vi "miniScanSelector.vi"(0 "X-Y-Z coordinates":T1 {"Apparent Frame Size" format="%#_6f"; "Original FOV (um)" format="%#_6f"; "Pixels per miniscan" format="%#_6f"; "Dwell Time per pixel" format="%#_6f"; "Resolution" format="%#_6f"; "ROI group ID" format="%#_6f"; "Laser Power (%)" format="%#_6f"; "Zoom" format="%#_6f"; "Frame Size" format="%#_6f"; "Number of lines" format="%#_6f"; "Composite ID" format="%#_6f"; "Angle (deg)" format="%#_6f"; "ROI Time (ns)" format="%#_6f"; "ROI ID" format="%#_6f"; "Pixels in ROI" format="%#_6f"; "ROI index" format="%#_6f"; "Z stop" format="%#_6f"; "Y stop" format="%#_6f"; "X stop" format="%#_6f"; "Z start" format="%#_6f"; "X start" format="%#_6f"; "Y start" format="%#_6f"}, 1 "index":i32, 2 "FrameSize":dbl, 3 "App. FrameSize":dbl, 5 "Main zoom":dbl) -> (14 "Norm X Start":dbl, 15 "Norm Y Start":dbl, 16 "Norm Z Start":dbl, 17 "Norm X Stop":dbl, 18 "Norm Y Stop":dbl, 19 "Norm Z Stop":dbl)   [LabVIEW 2020]
uses:
  User Interface/Visualisation/Functional Imaging Viewer/Typedefs/ROI parameters data type.ctl
panel:
  in  "Temporary offset (0)":dbl format="%#_13g"
  # "<--- For vertical miniscans only"
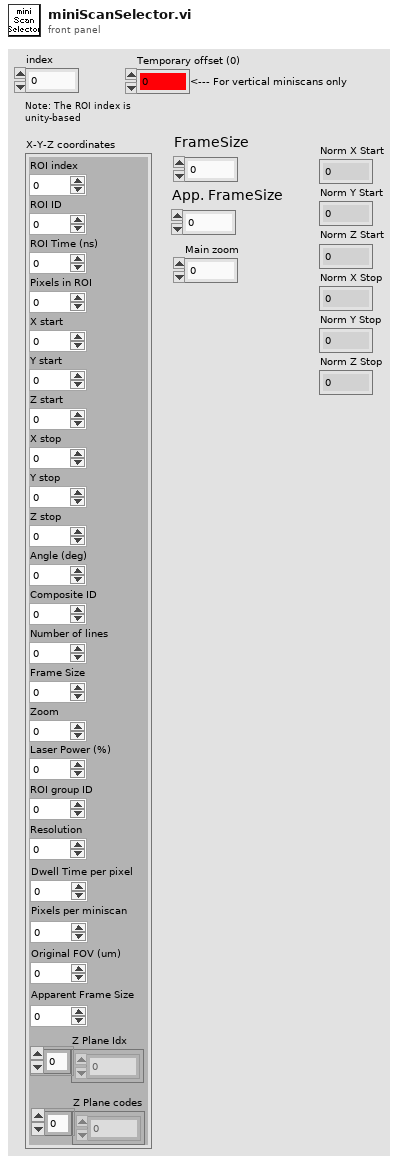
[diagram p1: front panel]
types:
  T1 = typedef "ROI parameters data type.ctl" = cluster{"ROI index":dbl, "ROI ID":dbl, "ROI Time (ns)":dbl, "Pixels in ROI":dbl, "X start":dbl, "Y start":dbl, "Z start":dbl, "X stop":dbl, "Y stop":dbl, "Z stop":dbl, "Angle (deg)":dbl, "Composite ID":dbl, "Number of lines":dbl, "Frame Size":dbl, "Zoom":dbl, "Laser Power (%)":dbl, "ROI group ID":dbl, "Resolution":dbl, "Dwell Time per pixel":dbl, "Pixels per miniscan":dbl, "Original FOV (um)":dbl, "Apparent Frame Size":dbl, "Z Plane Idx":i32[], "Z Plane codes":i32[]}
  T2 = typedef "Angle type.ctl" = enum16{"Horisontal (0 deg)", "Vertical (90 deg)", "Any other angle"}
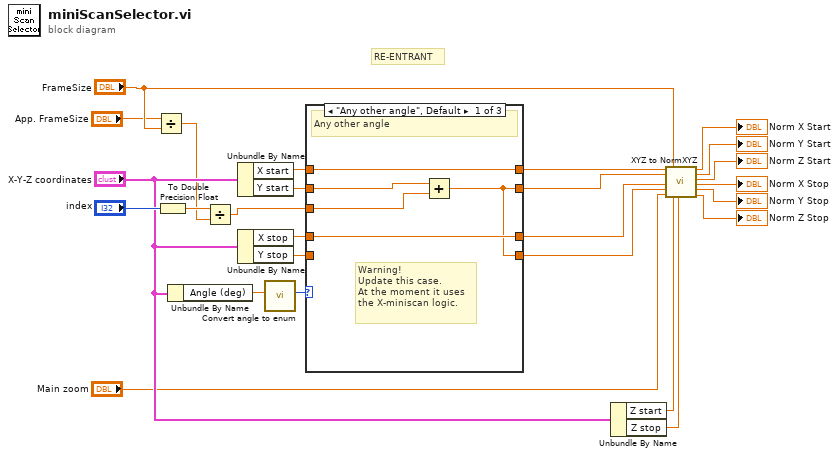
[diagram p0: block diagram]
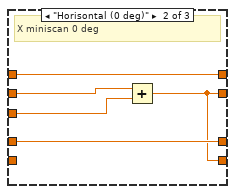
[diagram p2: hidden frame]
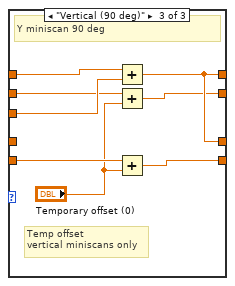
[diagram p3: hidden frame]
diagram:
  # "RE-ENTRANT"
  n1 = Divide(x="App. FrameSize", y="FrameSize") -> (x/y=w2:dbl)
  n2 = To Double Precision Float(number="index") -> (double precision float=w3:dbl)
  n3 = Unbundle By Name("X-Y-Z coordinates") -> ("Angle (deg)"=w8:dbl)
  n4 = Divide(x=w3, y=w2) -> (x/y=w1:dbl)
  n5 = Unbundle By Name("X-Y-Z coordinates") -> ("X start"=w25:dbl, "Y start"=w24:dbl)
  n6 = Unbundle By Name("X-Y-Z coordinates") -> ("X stop"=w23:dbl, "Y stop"=w22:dbl)
  n7 = call "Convert angle to enum.vi"("Angle"=w8) -> ("Miniscan angle"=w7:T2)  [unwired: 10 in]
  n8 = case shown="\"Any other angle\", Default" w7 {
    tunnel: [w31 w36 w43] -> w21
    tunnel: w25 -> [w31 w36 w42]
    tunnel: w24 -> [w28 w33 w41]
    tunnel: [w27 w32 w40] -> w20
    tunnel: w23 -> [w30 w35 _]
    tunnel: [w30 w35 w43] -> w19
    tunnel: w22 -> [_ _ w39]
    tunnel: [w27 w32 w38] -> w18
    tunnel: w1 -> [w29 w34 w44]
    frame "Any other angle", Default {
      # "Warning!\nUpdate this case.\nAt the moment it uses\nthe X-miniscan logic."
      # "Any other angle"
      n9 = Add(x=w28, y=w29) -> (x+y=w27:dbl)
    }
    frame "Horisontal (0 deg)" {
      # "X miniscan 0 deg"
      n10 = Add(x=w33, y=w34) -> (x+y=w32:dbl)
    }
    frame "Vertical (90 deg)" {
      # "Temp offset\nvertical miniscans only"
      # "Y miniscan 90 deg"
      n11 = Add(x=w42, y=w44) -> (x+y=w43:dbl)
      n12 = Add(x=w41, y="Temporary offset (0)") -> (x+y=w40:dbl)
      n13 = Add(x=w39, y="Temporary offset (0)") -> (x+y=w38:dbl)
    }
  }
  n14 = Unbundle By Name("X-Y-Z coordinates") -> ("Z start"=w17:dbl, "Z stop"=w16:dbl)
  n15 = call "XYZ to NormXYZ.vi"("X start"=w21, "Y start"=w20, "X stop"=w19, "Y stop"=w18, "Zoom (either ref or main zoom)"="Main zoom", "FrameSize"="FrameSize", "Z start"=w17, "Z stop"=w16) -> ("Norm X Start"=→"Norm X Start":dbl, "Norm Y Start"=→"Norm Y Start":dbl, "Norm Z Start"=→"Norm Z Start":dbl, "Norm X Stop"=→"Norm X Stop":dbl, "Norm Y Stop"=→"Norm Y Stop":dbl, "Norm Z Stop"=→"Norm Z Stop":dbl)  [unwired: 6 in]
